vi "FRONT_PANEL_14.vi"() -> ()   [LabVIEW 2022 SP3]
doc: "This application VI allows the user to set the desired parameters in the \n5800 / 5900 P / R. just select thevalues that you want to set the instrument to from the 5800 / 5900 user interface and click on the send to 5800 button."
uses:
  <vilib>/Instr/_visa.llb/VISA Configure Serial Port (Instr).vi
  PulserGlobals.vi
panel:
  out "Error Out":errorcluster
  in  "Error In":errorcluster
  in  "Puls mode":u16(ring)=3 items=["Half cycle positive", "Half cycle negegative", "Full cycle positive", "Full cycle negative"]
  in  "pulser ON/OFF":bool
  in  "remote echo":bool
  in  "internal trigger":bool
  in  "high gain (+ 15.5 dB)":bool
  in  "Freq. [MHz]":i16=40 min=5 max=50 step=1
  out "freq   string":string
  in  "Voltage [V]":i16=35 min=5 max=60 step=5
  out "String to write":string
  in  "Gain [dB]":i16=33 min=0 max=51 step=1
  in  "VISA Resource Name -  ASRL1::INSTR":refnum<visa-resource-name>="COM5"
  in  "ExitSendCmd":bool
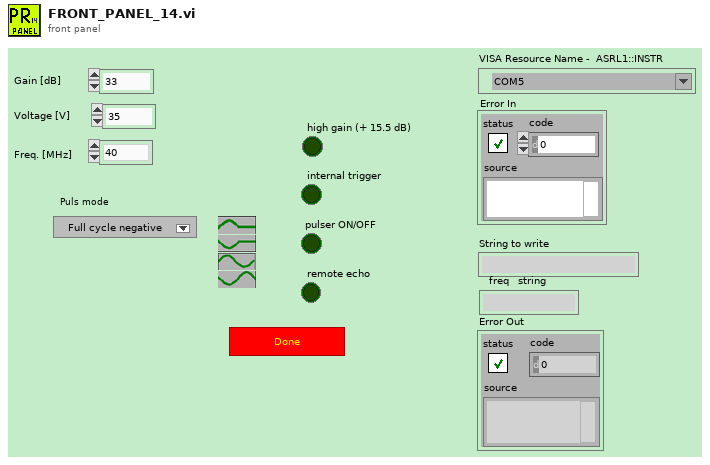
[diagram p1: front panel]
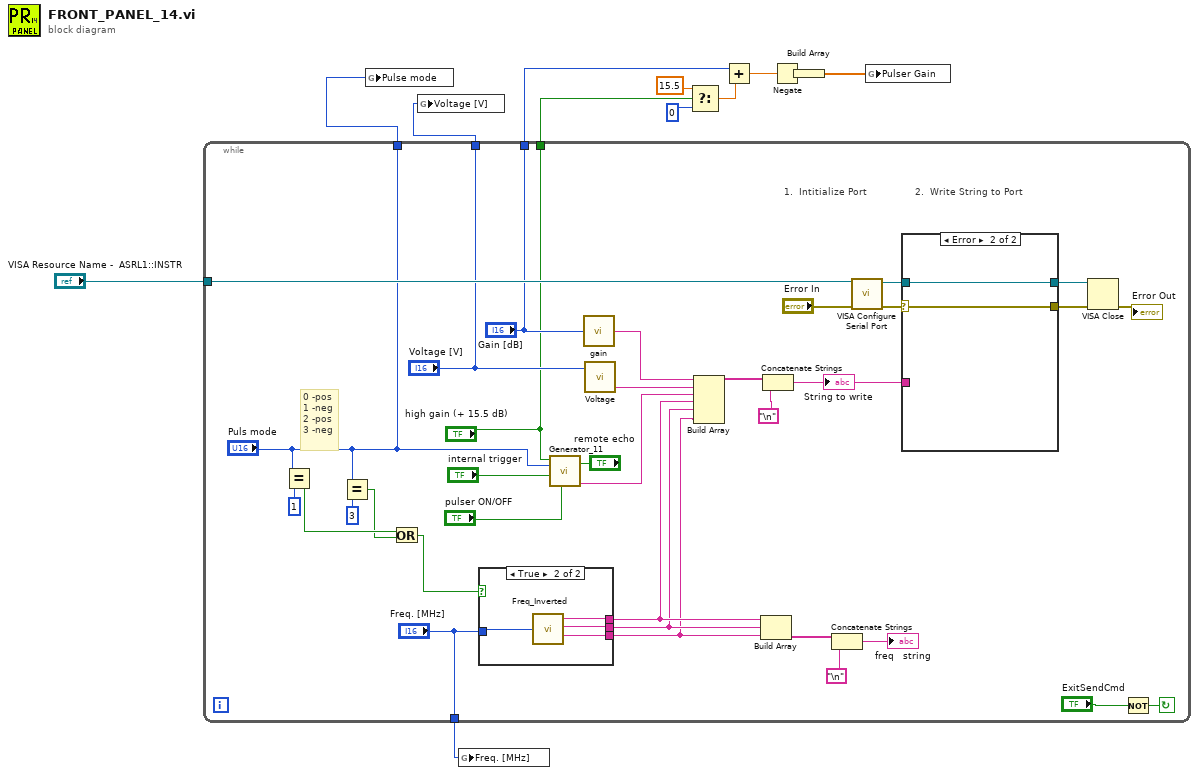
[diagram p0: block diagram]
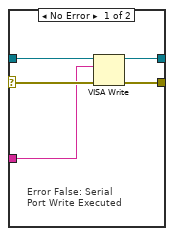
[diagram p2: hidden frame]
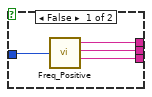
[diagram p3: hidden frame]
diagram:
  n1 = while {
    tunnel: "VISA Resource Name -  ASRL1::INSTR" -> [w21]
    tunnel: ["Puls mode"] -> w3
    tunnel: ["Voltage [V]"] -> w2
    tunnel: ["Freq. [MHz]"] -> w1
    tunnel: ["Gain [dB]"] -> w11
    tunnel: ["high gain (+ 15.5 dB)"] -> w7
    stop <- w46 continue-if-true
    # "1.  Intitialize Port"
    # "2.  Write String to Port"
    # "0 -pos\n1 -neg\n2 -pos\n3 -neg"
    n2 = Equal?(x="Puls mode", y=1) -> (x = y?=w32:bool)
    n3 = Equal?(x="Puls mode", y=3) -> (x = y?=w31:bool)
    n4 = Or(x=w32, y=w31) -> (x .or. y?=w30:bool)
    n5 = case shown="True" w30 {
      tunnel: [w57 w58] -> w20
      tunnel: [w56 w61] -> w19
      tunnel: [w55 w60] -> w18
      tunnel: "Freq. [MHz]" -> [w54 w59]
      frame False {
        n6 = call "Freq_Positive.vi"("enter freq [MHz]"=w54) -> ("T1 command  str"=w57:string, "T2 command  str"=w56:string, "T3 command  str"=w55:string)
      }
      frame True {
        n7 = call "Freq_Inverted.vi"("enter freq [MHz]"=w59) -> ("T1 command  str"=w58:string, "T2 command  str"=w61:string, "T3 command  str"=w60:string)
      }
    }
    n8 = call "Generator_11.vi"("pulser ON/OFF"="pulser ON/OFF", "remote echo"="remote echo", "internal trigger"="internal trigger", "Puls mode"="Puls mode", "high gain"="high gain (+ 15.5 dB)") -> ("Command_ str"=w29:string)  [unwired: 4 out]
    n9 = call "gain.vi"("gain"="Gain [dB]") -> ("Command_ str"=w42:string)
    n10 = call "Voltage.vi"("volt"="Voltage [V]") -> ("Command_ str"=w41:string)
    n11 = Build Array "Build Array"(w42, w41, w29, w20, w19, w18) -> (w43:string[])
    n12 = Build Array "Build Array"(w20, w19, w18) -> (w39:string[])
    n13 = Concatenate Strings(w43, "\n") -> (w22:string)
    "String to write" <- w22
    n14 = Concatenate Strings(w39, "\n") -> (→"freq   string":string)
    n15 = call-poly "VISA Configure Serial Port"("VISA resource name"=w21, "error in (no error)"="Error In") -> ("VISA resource name out"=w27:refnum<visa-resource-name>, "error out"=w26:errorcluster)  [unwired: 4 in, 8 out]
    n16 = case shown="Error" w26 {
      selector: w26 -> [w50 w52]
      tunnel: w27 -> [w51 w53]
      tunnel: [w49 w52] -> w23
      tunnel: [w48 w53] -> w24
      tunnel: w22 -> [w47 _]
      frame No Error {
        # "Error False: Serial\nPort Write Executed"
        n17 = VISA Write(VISA resource name=w51, write buffer=w47, error in (no error)=w50) -> (VISA resource name out=w48:refnum<visa-resource-name>, error out=w49:errorcluster)  [unwired: 1 out]
      }
      frame Error {
      }
    }
    n18 = VISA Close(VISA resource name=w24, error in (no error)=w23) -> (error out=→"Error Out":errorcluster)
    n19 = Not(x="ExitSendCmd") -> (.not. x?=w46:bool)
  }
  n20 = global write "PulserGlobals.vi" "Pulse mode"(w3) -> ()
  n21 = global write "PulserGlobals.vi" "Voltage [V]"(w2) -> ()
  n22 = global write "PulserGlobals.vi" "Freq. [MHz]"(w1) -> ()
  n23 = Select(t=15.5, s=w7, f=0) -> (s? t:f=w9:dbl)
  n24 = Add(x=w11, y=w9) -> (x+y=w10:dbl)
  n25 = Negate(x=w10) -> (-x=w5:dbl)
  n26 = Build Array(w5) -> (w4:dbl[])
  n27 = global write "PulserGlobals.vi" "Pulser Gain"(w4) -> ()
